vi "Encoder Rate Shooter.vi"() -> ()   [LabVIEW 2016]
panel:
  in  "5)(0073R R473":dbl
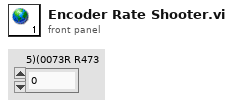
[diagram p1: front panel]
diagram:
